vi "Calculate BER (SubVI).vi"(1 "Original Bits":i8[](array[numeric]), 2 "Demod Bits":i8[](array[numeric])) -> (0 "BER":dbl)   [LabVIEW 2015]
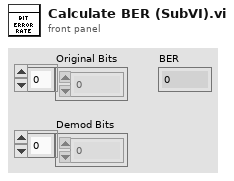
[diagram p1: front panel]
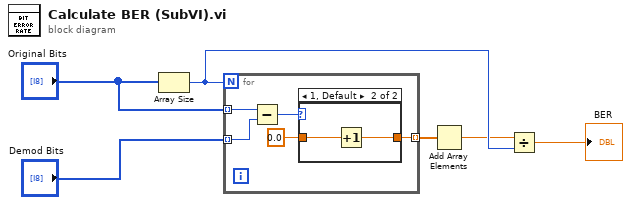
[diagram p0: block diagram]
diagram:
  n1 = Array Size(array="Original Bits") -> (size(s)=w6:i32)
  n2 = for {
    N: w6 -> [_]
    tunnel: "Original Bits" -> [w11] mode=indexing
    tunnel: "Demod Bits" -> [w10] mode=indexing
    tunnel: [w8] -> w3 mode=indexing
    n3 = Subtract(x=w11, y=w10) -> (x-y=w9:i8)
    n4 = case shown="1, Default" w9 {
      tunnel: 0.0 ("element") -> [_ w13]
      tunnel: [_ w12] -> w8
      frame 0 {
      }
      frame 1, Default {
        n5 = Increment(x=w13) -> (x+1=w12:dbl)
      }
    }
  }
  n6 = Add Array Elements(numeric array=w3) -> (sum=w4:dbl)
  n7 = Divide(x=w4, y=w6) -> (x/y=→"BER":dbl)
